vi "Redraw All Panels in Device List.vi"(8 "error in (no error)":errorcluster, 11 "Device List State":T1) -> (0 "error out":errorcluster, 3 "Device List State out":T1)   [LabVIEW 2015]
uses:
  Device List State.ctl
  Device/Device.lvclass
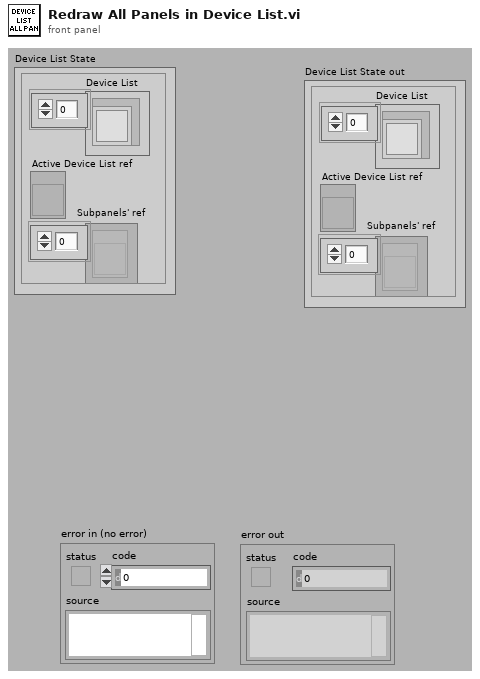
[diagram p1: front panel]
types:
  T1 = typedef "Device List State.ctl" = cluster{"Device List":refnum<class "Device.lvclass">[], "Active Device List ref":refnum<vi>, "Subpanels' ref":refnum<vi>[]}
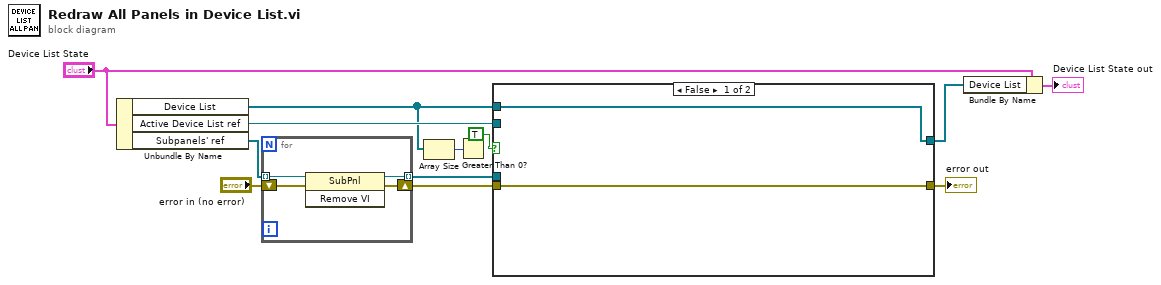
[diagram p0: block diagram]
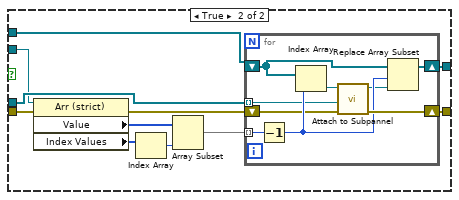
[diagram p2: hidden frame]
diagram:
  n1 = Unbundle By Name("Device List State") -> ("Device List"=w2:refnum<class "Device.lvclass">[], "Active Device List ref"=w4:refnum<vi>, "Subpanels' ref"=w7:refnum<vi>[])
  n2 = for {
    tunnel: w7 -> [w16] mode=indexing
    shift-right: [w14] -> w5
    shift-left: "error in (no error)" -> [w13]
    tunnel: [w15] -> w8 mode=indexing
    n3 = invoke class="SubPnl" method="Remove VI"(reference=w16, error in=w13) -> (reference out=w15:refnum<vi>, error out=w14:errorcluster)  [unwired: 1 in, 1 out]
  }
  n4 = Array Size(array=w2) -> (size(s)=w3:i32)
  n5 = Greater Than 0?(x=w3) -> ()  [unwired: 1 out]
  n6 = case shown="False" TRUE {
    tunnel: [w18 w28] -> w12
    tunnel: [w17 w27] -> w10
    tunnel: w8 -> [_ w23]
    tunnel: w2 -> [w17 w22]
    tunnel: w5 -> [w18 w21]
    tunnel: w4 -> [_ w19]
    frame False {
    }
    frame True {
      n7 = property class="Arr (strict)"(reference=w19, error in=w21) -> (error out=w20:errorcluster, "Value"=w26:u16[], "Index Values"=w25:u32[])  [unwired: 1 out]
      n8 = Index Array(array=w25) -> (element=w24:u32)  [unwired: 1 in]
      n9 = Array Subset(array=w26, index=w24) -> (w29:u16[])  [unwired: 1 in]
      n10 = for {
        tunnel: w23 -> [w31] mode=indexing
        shift-right: [w38] -> w28
        shift-left: w20 -> [w30]
        tunnel: w29 -> [w37] mode=indexing
        shift-right: [w35] -> w27
        shift-left: w22 -> [w36]
        n11 = Decrement(x=w37) -> (x-1=w33:u16)
        n12 = Index Array(array=w36, index=w33) -> (element=w34:refnum<class "Device.lvclass">)
        n13 = call "Attach to Subpannel.vi"("error in (no error)"=w30, "Sub Panel"=w31, "Device in"=w34) -> ("error out"=w38:errorcluster, "Device out"=w32:refnum<class "Device.lvclass">)  [unwired: 7 in]
        n14 = Replace Array Subset(array=w36, new element=w32, index=w33) -> (w35:refnum<class "Device.lvclass">[])
      }
    }
  }
  "error out" <- w12
  n15 = Bundle By Name(cluster="Device List State", "Device List"=w10) -> (→"Device List State out":T1)
